vi "Field Info to Cluster Item Info (Array).vi"(1 "Fields Info":T3[](array[typedef])) -> (0 "Cluster Items":T1[](array[typedef]))   [LabVIEW 2021]
uses:
  edt.lib/sqlite.lib/SQLite Field Info.ctl
  edt.lib/sqlite.lib/SQLite Data Type.ctl
  edt.lib/vi_script.lib/Cluster Item Info.ctl
  <vilib>/Utility/Data Type/Type Definitions/Data Type.ctl
  SQLite Data Type to LV Data Type.ctl
  <vilib>/Utility/Data Type/NI_Data Type.lvlib
  edt.lib/vi_script.lib/EDT VI Script.lvlib
  edt.lib/sqlite.lib/EDT SQLite+.lvlib
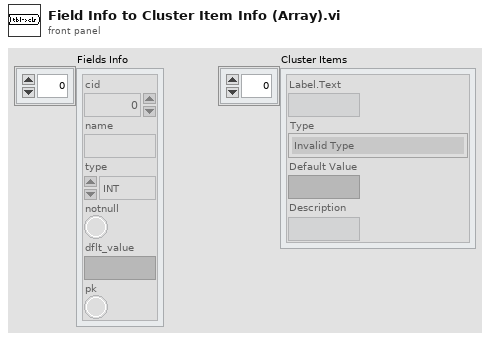
[diagram p1: front panel]
types:
  T1 = typedef "EDT VI Script.lvlib/Cluster Item Info.ctl" = cluster{"Label.Text":string, "Type":T2, "Default Value":variant, "Description":string}
  T2 = typedef "NI_Data Type.lvlib/Data Type.ctl" = enum8{"Invalid Type", "Void", "I8", "I16", "I32", "I64", "U8", "U16", "U32", "U64", "Single Float", "Double Float", "Extended Float", "Single Complex", "Double Complex", "Extended Complex", "Enum U8", "Enum U16", "Enum U32", "Enum U64", "Single Float With Unit", "Double Float With Unit", "Extended Float With Unit", "Single Complex with Unit", "Double Complex with Unit", "Extended Complex with Unit", "Boolean", "String", "Path", "Picture", "Tag", "Array", "Cluster", "Variant", "LV Variant", "Waveform", "Timestamp", "Digital Waveform", "Digital Data", "ExpressData", "Refnum", "External Data", "VI", "Poly VI", "LabVIEW Class Instance", "Fixed Point", "Set Collection", "Map Collection"}
  T3 = typedef "EDT SQLite+.lvlib/SQLite Field Info.ctl" = cluster{"cid":i32, "name":string, "type":T4, "notnull":bool, "dflt_value":variant, "pk":bool}
  T4 = typedef "EDT SQLite+.lvlib/SQLite Data Type.ctl" = enum16{"INT", "INTEGER", "TINYINT", "SMALLINT", "MEDIUMINT", "BIGINT", "UNSIGNED BIG INT", "INT2", "INT8", "CHARACTER", "VARCHAR", "VARYING CHARACTER", "NCHAR", "NATIVE CHARACTER", "NVARCHAR", "TEXT", "CLOB", "BLOB", "no datatype specified", "REAL", "DOUBLE", "DOUBLE PRECISION", "FLOAT", "NUMERIC", "DECIMAL", "BOOLEAN", "DATE", "DATETIME"}
  T5 = typedef "SQLite Data Type to LV Data Type.ctl" = map{T4, T2}
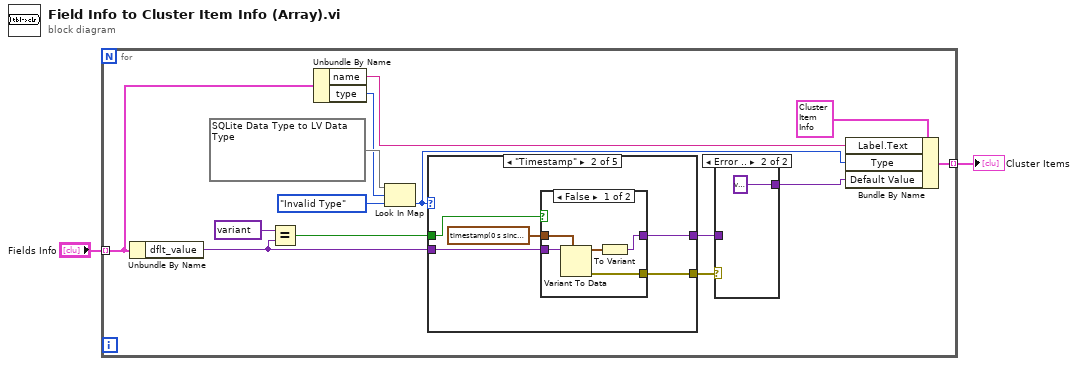
[diagram p0: block diagram]
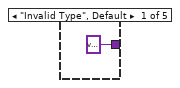
[diagram p3: hidden frame]
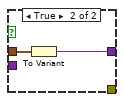
[diagram p4: hidden frame]
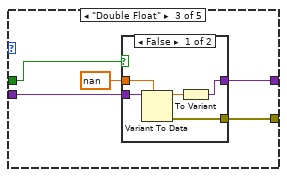
[diagram p5: hidden frame]
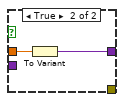
[diagram p6: hidden frame]
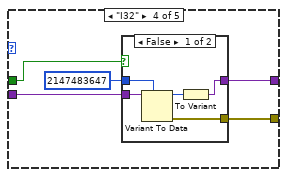
[diagram p7: hidden frame]
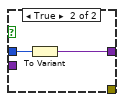
[diagram p8: hidden frame]
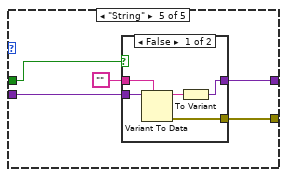
[diagram p9: hidden frame]
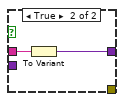
[diagram p10: hidden frame]
diagram:
  n1 = for {
    tunnel: [w12] -> w2 mode=indexing
    tunnel: "Fields Info" -> [w6] mode=indexing
    n2 = Unbundle By Name(w6) -> ("dflt_value"=w5:variant)
    n3 = Equal?(x=variant ("dflt_value"), y=w5) -> (x = y?=w3:bool)
    n4 = Unbundle By Name(w6) -> ("name"=w11:string, "type"=w9:T4)
    n5 = Look In Map(map=T5 {enum."INT"=enum."I32", enum."INTEGER"=enum."I32", enum."TINYINT"=enum."I32", enum."SMALLINT"=enum."I32", enum."MEDIUMINT"=enum."I32", enum."BIGINT"=enum."I32", enum."UNSIGNED BIG INT"=enum."I32", enum."INT2"=enum."I32", enum."INT8"=enum."I32", enum."CHARACTER"=enum."String", enum."VARCHAR"=enum."String", enum."VARYING CHARACTER"=enum."String", enum."NCHAR"=enum."String", enum."NATIVE CHARACTER"=enum."String", enum."NVARCHAR"=enum."String", enum."TEXT"=enum."String", enum."CLOB"=enum."String", enum."BLOB"=enum."String", enum."no datatype specified"=enum."String", enum."REAL"=enum."Double Float", enum."DOUBLE"=enum."Double Float", enum."DOUBLE PRECISION"=enum."Double Float", enum."FLOAT"=enum."Double Float", enum."NUMERIC"=enum."Double Float", enum."DECIMAL"=enum."Double Float", enum."BOOLEAN"=enum."I32", enum."DATE"=enum."Timestamp", enum."DATETIME"=enum."Timestamp"} ("SQLite Data Type to LV Data Type"), key=w9, default value=Data_Type."Invalid Type" ("type")) -> (value=w7:T2)  [unwired: 1 out]
    n6 = case shown="\"Timestamp\"" w7 {
      tunnel: w5 -> [_ w24 w36 w48 w60]
      tunnel: [variant ("Variant") w22 w35 w47 w59] -> w15
      tunnel: [_ w21 w33 w45 w57] -> w16
      tunnel: w3 -> [_ w20 w32 w44 w56]
      frame "Invalid Type", Default {
      }
      frame "Timestamp" {
        n7 = case shown="False" w20 {
          tunnel: [w28 w31] -> w22
          tunnel: w24 -> [w29 _]
          tunnel: timestamp(0 s since 1904-01-01) ("Time Stamp") -> [w26 w30]
          tunnel: [w25 _] -> w21
          frame False {
            n8 = Variant To Data(type=w26, Variant=w29) -> (data=w27:timestamp, error out=w25:errorcluster)  [unwired: 1 in]
            n9 = To Variant(anything=w27) -> (Variant=w28:variant)
          }
          frame True {
            n10 = To Variant(anything=w30) -> (Variant=w31:variant)
          }
        }
      }
      frame "Double Float" {
        n11 = case shown="False" w32 {
          tunnel: [w40 w43] -> w35
          tunnel: w36 -> [w41 _]
          tunnel: nan -> [w38 w42]
          tunnel: [w37 _] -> w33
          frame False {
            n12 = Variant To Data(type=w38, Variant=w41) -> (data=w39:dbl, error out=w37:errorcluster)  [unwired: 1 in]
            n13 = To Variant(anything=w39) -> (Variant=w40:variant)
          }
          frame True {
            n14 = To Variant(anything=w42) -> (Variant=w43:variant)
          }
        }
      }
      frame "I32" {
        n15 = case shown="False" w44 {
          tunnel: [w52 w55] -> w47
          tunnel: w48 -> [w53 _]
          tunnel: 2147483647 -> [w50 w54]
          tunnel: [w49 _] -> w45
          frame False {
            n16 = Variant To Data(type=w50, Variant=w53) -> (data=w51:i32, error out=w49:errorcluster)  [unwired: 1 in]
            n17 = To Variant(anything=w51) -> (Variant=w52:variant)
          }
          frame True {
            n18 = To Variant(anything=w54) -> (Variant=w55:variant)
          }
        }
      }
      frame "String" {
        n19 = case shown="False" w56 {
          tunnel: [w64 w67] -> w59
          tunnel: w60 -> [w65 _]
          tunnel: "" -> [w62 w66]
          tunnel: [w61 _] -> w57
          frame False {
            n20 = Variant To Data(type=w62, Variant=w65) -> (data=w63:string, error out=w61:errorcluster)  [unwired: 1 in]
            n21 = To Variant(anything=w63) -> (Variant=w64:variant)
          }
          frame True {
            n22 = To Variant(anything=w66) -> (Variant=w67:variant)
          }
        }
      }
    }
    n23 = case shown="Error .." w16 {
      tunnel: w15 -> [w17 _]
      tunnel: [w17 variant ("Variant")] -> w14
      frame No Error {
      }
      frame Error {
      }
    }
    n24 = Bundle By Name(cluster=T1 {"Label.Text"="", "Type"=enum."Invalid Type", "Default Value"=variant(string ""), "Description"=""} ("Cluster Item"), "Label.Text"=w11, "Type"=w7, "Default Value"=w14) -> (w12:T1)
  }
  "Cluster Items" <- w2
